vi "SetControllerDependency.vi"(8 "error in (no error)":errorcluster, 10 "Measurement":refnum<class "Measurement.lvclass">, 11 "Measurement.UI in":refnum<class "Measurement.UI.lvclass">) -> (0 "error out":errorcluster, 3 "Measurement.UI out":refnum<class "Measurement.UI.lvclass">)   [LabVIEW 2017, in "Measurement.UI.lvclass"]
uses:
  Measurement.UI.lvclass
  Measurement/Measurement.lvclass
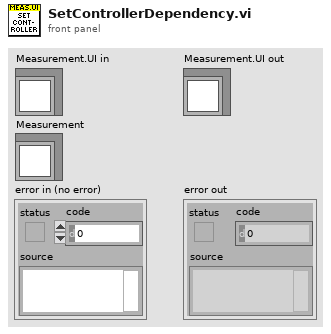
[diagram p1: front panel]
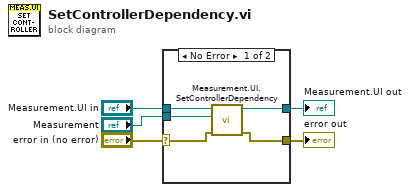
[diagram p0: block diagram]
diagram:
  n1 = case shown="No Error" "error in (no error)" {
    selector: "error in (no error)" -> [w8 w12]
    tunnel: [w6 w12] -> w4
    tunnel: [w7 w11] -> w2
    tunnel: "Measurement.UI in" -> [w10 w11]
    tunnel: "Measurement" -> [w9 _]
    frame No Error {
      n2 = call-dynamic "Measurement.UI.SetControllerDependency.vi"("error in (no error)"=w8, "Measurement"=w9, "Measurement.UI in"=w10) -> ("error out"=w6:errorcluster, "Measurement.UI out"=w7:refnum<class "Measurement.UI.lvclass">)  [unwired: 7 in]
    }
    frame Error {
    }
  }
  "error out" <- w4
  "Measurement.UI out" <- w2
